vi "Get_Sweep_Stop_Frequency.vi"(8 "error in (no error)":errorcluster, 11 ".NET Reference in":refnum<k24>) -> (0 "error out":errorcluster, 2 "stopfreq":dbl, 3 ".NET Reference out":refnum<k24>)   [LabVIEW 2017]
uses:
  D:/test/FULLband-sts/Fullband_Sample/DLL/InstrumentDLL.dll
  DLL/InstrumentDLL.dll
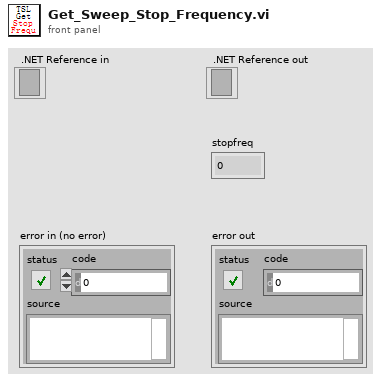
[diagram p1: front panel]
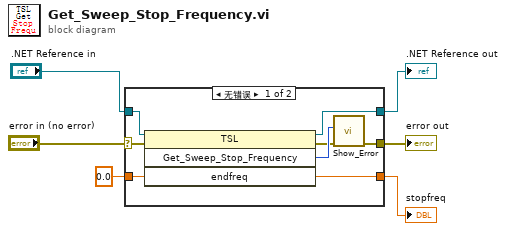
[diagram p0: block diagram]
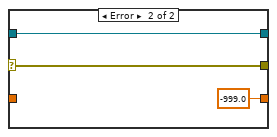
[diagram p2: hidden frame]
diagram:
  n1 = case shown="无错误" "error in (no error)" {
    selector: "error in (no error)" -> [w7 w16]
    tunnel: [w8 w16] -> w6
    tunnel: [w14 w15] -> w5
    tunnel: ".NET Reference in" -> [w13 w15]
    tunnel: [w12 -999.0 ("endfreq")] -> w3
    tunnel: 0.0 ("startfreq") -> [w11 _]
    frame No Error {
      n2 = invoke on="调用节点" class="TSL" method="Get_Sweep_Stop_Frequency"(reference=w13, error in=w7, "endfreq"=w11) -> (reference out=w14:refnum<k24>, error out=w9:errorcluster, "Get_Sweep_Stop_Frequency"=w10:i32, "endfreq"=w12:dbl)  [unwired: 1 in]
      n3 = call "Show_Error.vi"("error in (no error)"=w9, "Error"=w10) -> ("error out"=w8:errorcluster)  [unwired: 9 in]
    }
    frame Error {
    }
  }
  "error out" <- w6
  ".NET Reference out" <- w5
  "stopfreq" <- w3
